vi "Settings.vi"(8 "ErrorArray":errorcluster[](array[cluster])) -> (0 "ErrorArray":errorcluster[](array[cluster]))   [LabVIEW 2014, in "Framework.lvlib" / "Config.lvclass"]
uses:
  Config.lvclass
  Typedefs/Logging.ctl
  Typedefs/eLogLvl.ctl
  Typedefs/RootDir.ctl
  Typedefs/clSettingsRefs.ctl
  Config.lvclass/Config.ctl
  Accessors/Write Logging.vi
  Read Logging.vi
  Accessors/Read PARTF Root Directory.vi
  Accessors/Write PARTF Root Directory.vi
  Accessors/Read ConfigFilePath.vi
  <vilib>/Utility/config.llb/NI_LVConfig.lvlib
  <userlib>/NIST/NISTErrorLib/NISTErrorLib.lvlib
panel:
  in  "PARTF Data Directory":T1
  in  "Logging":T2={"eLogLvl"=enum."Normal", "Log File Path"=path "C:/Users/gra1/AppData/Local/Framework/Framework.log", "btnLogFile"=FALSE}
  in  "btnCancel":bool
  in  "btnDone":bool
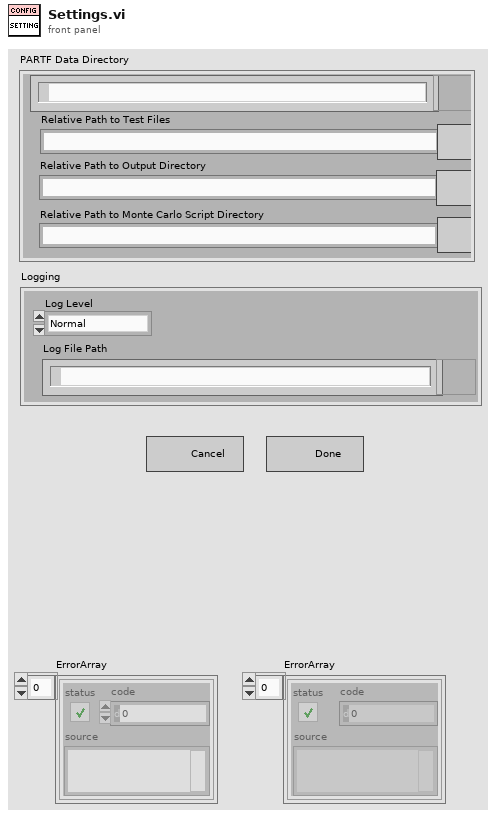
[diagram p1: front panel]
types:
  T1 = typedef "Framework.lvlib/Config.lvclass/RootDir.ctl" = cluster{"pathRootDir":path, "btnOutPath":bool, "OutDir":string, "btnOpenOutputDir":bool, "ScriptDir":string, "btnOpenScriptDir":bool, "TestDir":string, "btnOpenTestDir":bool}
  T2 = typedef "Framework.lvlib/Config.lvclass/Logging.ctl" = cluster{"eLogLvl":T3, "Log File Path":path, "btnLogFile":bool}
  T3 = typedef "Framework.lvlib/Config.lvclass/eLogLvl.ctl" = enum16{"Normal", "Verbose", "None"}
  T4 = typedef "Framework.lvlib/Config.lvclass/clSettingsRefs.ctl" = cluster{"PARTF Data Directory":refnum<vi>, "Logging":refnum<vi>}
  T5 = typedef "NI_LVConfig.lvlib/Config Data RefNum.ctl" = refnum<k1>
  T6 = cluster{"pathRootDir":path, "OutDir":string, "ScriptDir":string, "TestDir":string}
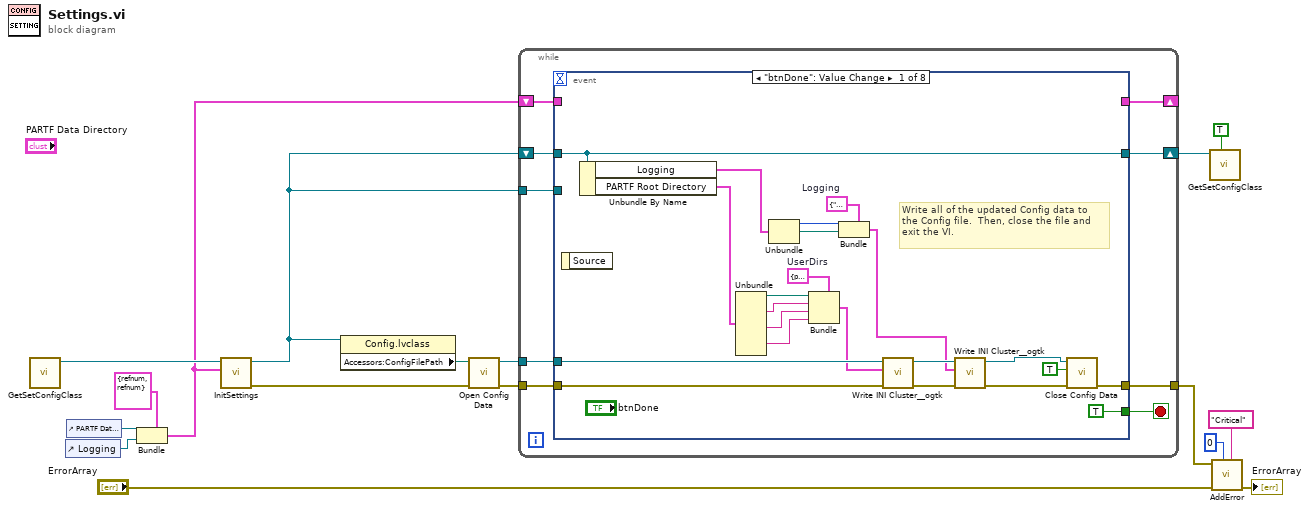
[diagram p0: block diagram]
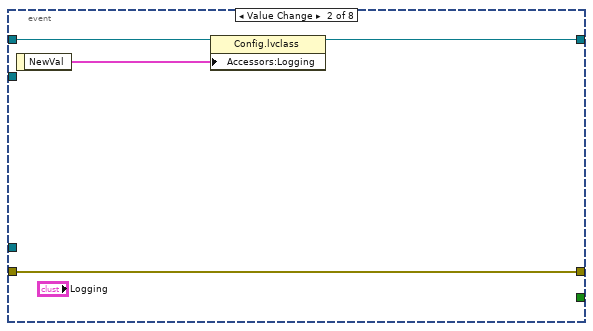
[diagram p2: hidden frame]
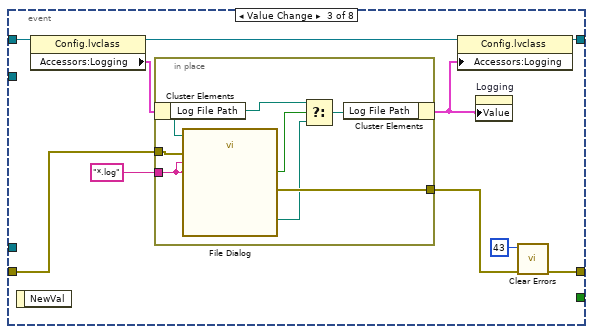
[diagram p3: hidden frame]
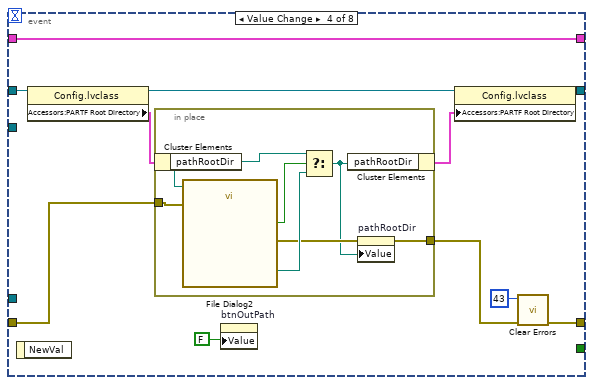
[diagram p4: hidden frame]
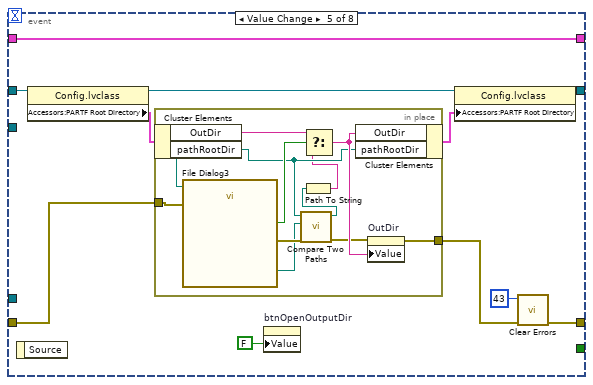
[diagram p5: hidden frame]
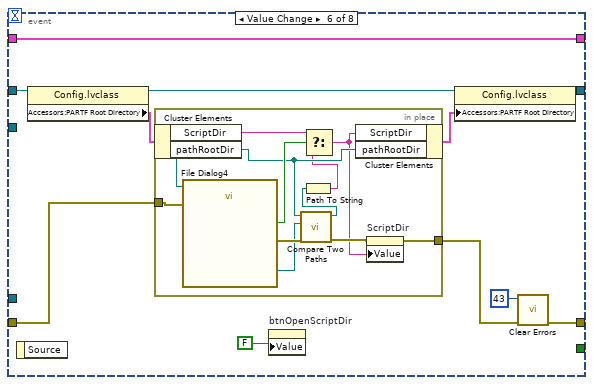
[diagram p6: hidden frame]
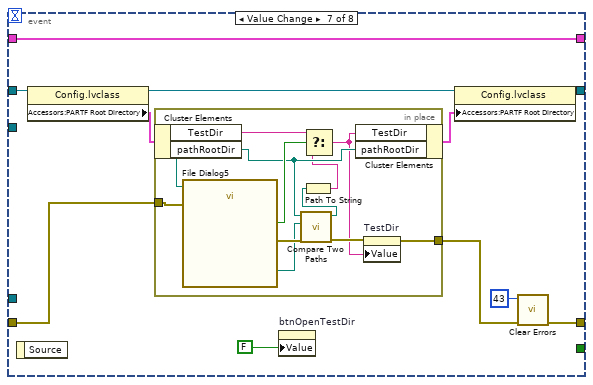
[diagram p7: hidden frame]
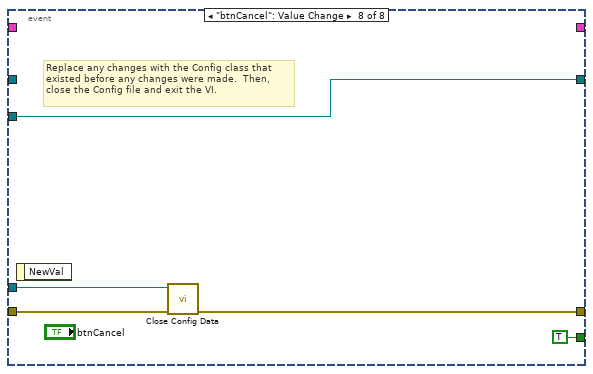
[diagram p8: hidden frame]
diagram:
  n1 = call "GetSetConfigClass.vi"() -> ("Ref out"=w4:refnum<class "Config.lvclass">)  [unwired: 11 in]
  n2 = control-ref of="Logging"() -> (w6:refnum<vi>)
  n3 = control-ref of="PARTF Data Directory"() -> (w7:refnum<vi>)
  n4 = Bundle(cluster=T4 {"PARTF Data Directory"=refnum, "Logging"=refnum} ("SettingRefs"), "PARTF Data Directory"=w7, "Logging"=w6) -> (w1:T4)
  n5 = call "InitSettings.vi"("refs"=w1, "Config"=w4) -> ("error out"=w2:errorcluster, "Config"=w3:refnum<class "Config.lvclass">)  [unwired: 8 in]
  n6 = property class="Config.lvclass"(reference=w3) -> ("Accessors:ConfigFilePath"=w14:path)  [unwired: 1 in, 2 out]
  n7 = call <vilib>:"Open Config Data.vi"("error in (no error)"=w2, "configuration file path"=w14) -> ("error out"=w16:errorcluster, "refnum"=w15:T5)  [unwired: 7 in, 1 out]
  n8 = while {
    tunnel: w16 -> [w26]
    tunnel: [w24] -> w13
    tunnel: w15 -> [w23]
    shift-right: [w22] -> w8
    shift-left: w3 -> [w21]
    tunnel: w3 -> [w20]
    shift-right: [w18] -> _
    shift-left: w1 -> [w19]
    stop <- w25 stop-if-true
    n9 = event shown="[0] \"btnDone\": Value Change" {
      selector: _ -> [_ _ _ _ _ _ _ _]
      dyn-events: _ -> [_ _ _ _ _ _ _ _]
      timeout: _ -> [_ _ _ _ _ _ _ _]
      tunnel: w21 -> [w39 w52 w62 w80 w98 w120 w142 _]
      tunnel: [w39 w51 w59 w77 w95 w117 w139 w154] -> w22
      tunnel: w26 -> [w44 w49 w58 w76 w94 w116 w138 w158]
      tunnel: [w48 w49 w56 w74 w92 w114 w136 w156] -> w24
      tunnel: [TRUE _ _ _ _ _ _ TRUE] -> w25
      tunnel: w23 -> [w45 _ _ _ _ _ _ w155]
      tunnel: w20 -> [_ _ _ _ _ _ _ w154]
      tunnel: w19 -> [_ _ _ w71 w89 w111 w133 _]
      tunnel: [_ _ _ w71 w89 w111 w133 _] -> w18
      event "btnDone": Value Change {
        w33 = T6 {"pathRootDir"=path "", "OutDir"="", "ScriptDir"="", "TestDir"=""}  # UserDirs
        w35 = cluster{"eLogLvl":T3, "Log File Path":path} {"eLogLvl"=enum."Normal", "Log File Path"=path ""}  # Logging
        # "Write all of the updated Config data to \nthe Config file.  Then, close the file and\nexit the VI."
        n10 = event-data() -> ()  [unwired: 1 in, 1 out]
        n11 = Unbundle By Name(w39) -> ("Logging"=w36:T2, "PARTF Root Directory"=w28:T1)
        n12 = Unbundle(w28) -> ("pathRootDir"=w29:path, "OutDir"=w30:string, "ScriptDir"=w31:string, "TestDir"=w32:string)  [unwired: 4 out]
        n13 = Unbundle(w36) -> ("eLogLvl"=w38:T3, "Log File Path"=w37:path)  [unwired: 1 out]
        n14 = Bundle(cluster=w33, "pathRootDir"=w29, "OutDir"=w30, "ScriptDir"=w31, "TestDir"=w32) -> (w27:T6)
        n15 = Bundle(cluster=w35, "eLogLvl"=w38, "Log File Path"=w37) -> (w34:cluster{"eLogLvl":T3, "Log File Path":path})
        n16 = call <userlib>:"Write INI Cluster__ogtk.vi"("error in (no error)"=w44, "INI Fomatted Cluster"=w27, "refnum"=w45) -> ("error out"=w43:errorcluster, "dup refnum"=w41:T5)  [unwired: 7 in]
        n17 = call <userlib>:"Write INI Cluster__ogtk.vi"("error in (no error)"=w43, "INI Fomatted Cluster"=w34, "refnum"=w41) -> ("error out"=w42:errorcluster, "dup refnum"=w40:T5)  [unwired: 7 in]
        n18 = call <vilib>:"Close Config Data.vi"("error in (no error)"=w42, "write file if changed (T)"=TRUE, "refnum"=w40) -> ("error out"=w48:errorcluster)  [unwired: 7 in, 1 out]
      }
      event Value Change {
        n19 = event-data() -> ("NewVal"=w50:T2)  [unwired: 1 in]
        n20 = property class="Config.lvclass"(reference=w52, "Accessors:Logging"=w50) -> (reference out=w51:refnum<class "Config.lvclass">)  [unwired: 1 in, 1 out]
      }
      event Value Change {
        n21 = event-data() -> ()  [unwired: 1 in, 1 out]
        n22 = property class="Config.lvclass"(reference=w62) -> (reference out=w60:refnum<class "Config.lvclass">, "Accessors:Logging"=w61:T2)  [unwired: 1 in, 1 out]
        n23 = in-place {
          in-place-border: [w69] -> w57
          in-place-border: w58 -> [w68]
          in-place-border: "*.log" -> [w63]
          n24 = in-place-cluster #1(w61) -> ("Log File Path"=w66:path)
          n25 = call "File Dialog"("start path"=w66, "error in"=w68, "pattern (all files)"=w63, "pattern label"=w63) -> ("selected path"=w65:path, "cancelled"=w67:bool, "error out"=w69:errorcluster)  [unwired: 8 in, 1 out]
          n26 = Select(t=w66, s=w67, f=w65) -> (s? t:f=w64:path)
          n27 = in-place-cluster #1("Log File Path"=w64) -> (w54:T2)
        }
        n28 = property class="Config.lvclass"(reference=w60, "Accessors:Logging"=w54) -> (reference out=w59:refnum<class "Config.lvclass">)  [unwired: 1 in, 1 out]
        n29 = property on="Logging" class="Clust"("Value"=w54) -> ()  [unwired: 2 in, 2 out]
        n30 = call <vilib>:"Clear Errors.vi"("error in (no error)"=w57, "specific error code to clear (0: all)"=43) -> ("error out"=w56:errorcluster)  [unwired: 4 in, 1 out]
      }
      event Value Change {
        n31 = event-data() -> ()  [unwired: 1 in, 1 out]
        n32 = property class="Config.lvclass"(reference=w80) -> (reference out=w78:refnum<class "Config.lvclass">, "Accessors:PARTF Root Directory"=w79:T1)  [unwired: 1 in, 1 out]
        n33 = in-place {
          in-place-border: [w82] -> w75
          in-place-border: w76 -> [w87]
          n34 = in-place-cluster #2(w79) -> ("pathRootDir"=w85:path)
          n35 = call "File Dialog2"("start path"=w85, "error in"=w87) -> ("selected path"=w84:path, "cancelled"=w86:bool, "error out"=w83:errorcluster)  [unwired: 10 in, 1 out]
          n36 = Select(t=w85, s=w86, f=w84) -> (s? t:f=w81:path)
          n37 = in-place-cluster #2("pathRootDir"=w81) -> (w72:T1)
          n38 = property on="pathRootDir" class="Path"(error in=w83, "Value"=w81) -> (error out=w82:errorcluster)  [unwired: 1 in, 1 out]
        }
        n39 = property on="btnOutPath" class="Bool (strict)"("Value"=FALSE) -> ()  [unwired: 2 in, 2 out]
        n40 = property class="Config.lvclass"(reference=w78, "Accessors:PARTF Root Directory"=w72) -> (reference out=w77:refnum<class "Config.lvclass">)  [unwired: 1 in, 1 out]
        n41 = call <vilib>:"Clear Errors.vi"("error in (no error)"=w75, "specific error code to clear (0: all)"=43) -> ("error out"=w74:errorcluster)  [unwired: 4 in, 1 out]
      }
      event Value Change {
        n42 = event-data() -> ()  [unwired: 1 in, 1 out]
        n43 = property class="Config.lvclass"(reference=w98) -> (reference out=w96:refnum<class "Config.lvclass">, "Accessors:PARTF Root Directory"=w97:T1)  [unwired: 1 in, 1 out]
        n44 = in-place {
          in-place-border: [w105] -> w93
          in-place-border: w94 -> [w109]
          n45 = in-place-cluster #3(w97) -> ("OutDir"=w107:string, "pathRootDir"=w102:path)
          n46 = call "File Dialog3"("start path"=w102, "error in"=w109) -> ("selected path"=w101:path, "cancelled"=w108:bool, "error out"=w104:errorcluster)  [unwired: 10 in, 1 out]
          n47 = call <vilib>:"Compare Two Paths.vi"("error in (no error)"=w104, "Path 2"=w101, "Path 1"=w102) -> ("error out"=w103:errorcluster, "Relative Path from 1 to 2"=w100:path)  [unwired: 5 in, 2 out]
          n48 = Path To String(path=w100) -> (string=w99:string)
          n49 = Select(t=w107, s=w108, f=w99) -> (s? t:f=w106:string)
          n50 = in-place-cluster #3("OutDir"=w106, "pathRootDir"=w102) -> (w90:T1)
          n51 = property on="OutDir" class="Str"(error in=w103, "Value"=w106) -> (error out=w105:errorcluster)  [unwired: 1 in, 1 out]
        }
        n52 = property on="btnOpenOutputDir" class="Bool (strict)"("Value"=FALSE) -> ()  [unwired: 2 in, 2 out]
        n53 = property class="Config.lvclass"(reference=w96, "Accessors:PARTF Root Directory"=w90) -> (reference out=w95:refnum<class "Config.lvclass">)  [unwired: 1 in, 1 out]
        n54 = call <vilib>:"Clear Errors.vi"("error in (no error)"=w93, "specific error code to clear (0: all)"=43) -> ("error out"=w92:errorcluster)  [unwired: 4 in, 1 out]
      }
      event Value Change {
        n55 = event-data() -> ()  [unwired: 1 in, 1 out]
        n56 = property class="Config.lvclass"(reference=w120) -> (reference out=w118:refnum<class "Config.lvclass">, "Accessors:PARTF Root Directory"=w119:T1)  [unwired: 1 in, 1 out]
        n57 = in-place {
          in-place-border: [w123] -> w115
          in-place-border: w116 -> [w131]
          n58 = in-place-cluster #4(w119) -> ("ScriptDir"=w129:string, "pathRootDir"=w127:path)
          n59 = call "File Dialog4"("start path"=w127, "error in"=w131) -> ("selected path"=w126:path, "cancelled"=w130:bool, "error out"=w128:errorcluster)  [unwired: 10 in, 1 out]
          n60 = call <vilib>:"Compare Two Paths.vi"("error in (no error)"=w128, "Path 2"=w126, "Path 1"=w127) -> ("error out"=w122:errorcluster, "Relative Path from 1 to 2"=w125:path)  [unwired: 5 in, 2 out]
          n61 = Path To String(path=w125) -> (string=w124:string)
          n62 = Select(t=w129, s=w130, f=w124) -> (s? t:f=w121:string)
          n63 = in-place-cluster #4("ScriptDir"=w121, "pathRootDir"=w127) -> (w112:T1)
          n64 = property on="ScriptDir" class="Str"(error in=w122, "Value"=w121) -> (error out=w123:errorcluster)  [unwired: 1 in, 1 out]
        }
        n65 = property on="btnOpenScriptDir" class="Bool (strict)"("Value"=FALSE) -> ()  [unwired: 2 in, 2 out]
        n66 = property class="Config.lvclass"(reference=w118, "Accessors:PARTF Root Directory"=w112) -> (reference out=w117:refnum<class "Config.lvclass">)  [unwired: 1 in, 1 out]
        n67 = call <vilib>:"Clear Errors.vi"("error in (no error)"=w115, "specific error code to clear (0: all)"=43) -> ("error out"=w114:errorcluster)  [unwired: 4 in, 1 out]
      }
      event Value Change {
        n68 = event-data() -> ()  [unwired: 1 in, 1 out]
        n69 = property class="Config.lvclass"(reference=w142) -> (reference out=w140:refnum<class "Config.lvclass">, "Accessors:PARTF Root Directory"=w141:T1)  [unwired: 1 in, 1 out]
        n70 = in-place {
          in-place-border: [w145] -> w137
          in-place-border: w138 -> [w153]
          n71 = in-place-cluster #5(w141) -> ("TestDir"=w151:string, "pathRootDir"=w149:path)
          n72 = call "File Dialog5"("start path"=w149, "error in"=w153) -> ("selected path"=w148:path, "cancelled"=w152:bool, "error out"=w150:errorcluster)  [unwired: 10 in, 1 out]
          n73 = call <vilib>:"Compare Two Paths.vi"("error in (no error)"=w150, "Path 2"=w148, "Path 1"=w149) -> ("error out"=w144:errorcluster, "Relative Path from 1 to 2"=w147:path)  [unwired: 5 in, 2 out]
          n74 = Path To String(path=w147) -> (string=w146:string)
          n75 = Select(t=w151, s=w152, f=w146) -> (s? t:f=w143:string)
          n76 = in-place-cluster #5("TestDir"=w143, "pathRootDir"=w149) -> (w134:T1)
          n77 = property on="TestDir" class="Str"(error in=w144, "Value"=w143) -> (error out=w145:errorcluster)  [unwired: 1 in, 1 out]
        }
        n78 = property on="btnOpenTestDir" class="Bool (strict)"("Value"=FALSE) -> ()  [unwired: 2 in, 2 out]
        n79 = property class="Config.lvclass"(reference=w140, "Accessors:PARTF Root Directory"=w134) -> (reference out=w139:refnum<class "Config.lvclass">)  [unwired: 1 in, 1 out]
        n80 = call <vilib>:"Clear Errors.vi"("error in (no error)"=w137, "specific error code to clear (0: all)"=43) -> ("error out"=w136:errorcluster)  [unwired: 4 in, 1 out]
      }
      event "btnCancel": Value Change {
        # "Replace any changes with the Config class that\nexisted before any changes were made.  Then,\nclose the Config file and exit the VI."
        n81 = event-data() -> ()  [unwired: 1 in, 1 out]
        n82 = call <vilib>:"Close Config Data.vi"("error in (no error)"=w158, "refnum"=w155) -> ("error out"=w156:errorcluster)  [unwired: 8 in, 1 out]
      }
    }
  }
  n83 = call "GetSetConfigClass.vi"("Set (f)"=TRUE, "Ref in"=w8) -> ()  [unwired: 9 in, 1 out]
  n84 = call <userlib>:"AddError.vi"("Severity"="Critical", "Priority"=u8 0, "ErrorArray"="ErrorArray", "error in (no error)"=w13) -> ("ErrorArray"=→"ErrorArray":errorcluster[])  [unwired: 6 in, 1 out]
